vi "R-peak_detection_V2.vi"(9 "Cooldown in":i64, 10 "Threshold":dbl, 11 "ECG_vector":dbl[](array[numeric])) -> (1 "Cooldown out":i64, 3 "Rpeak_detected":bool)   [LabVIEW 2022 SP3]
uses:
  <vilib>/Analysis/NI_AALBase.lvlib
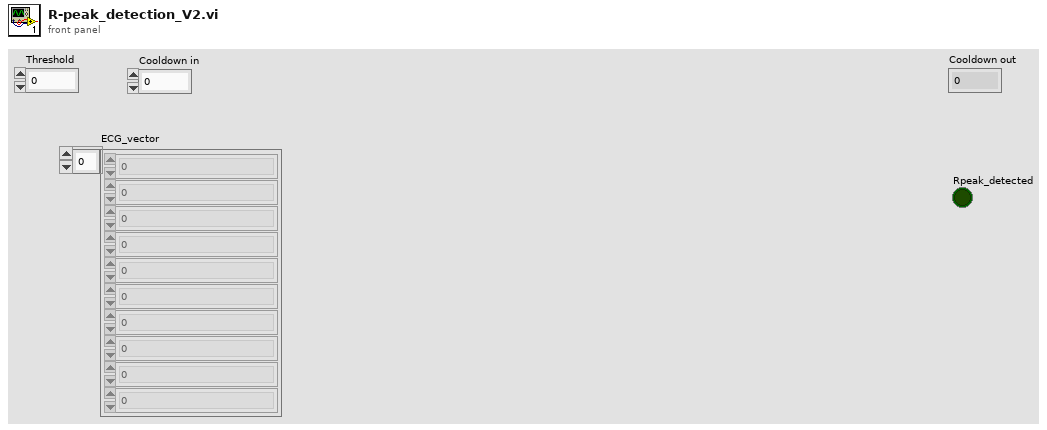
[diagram p1: front panel]
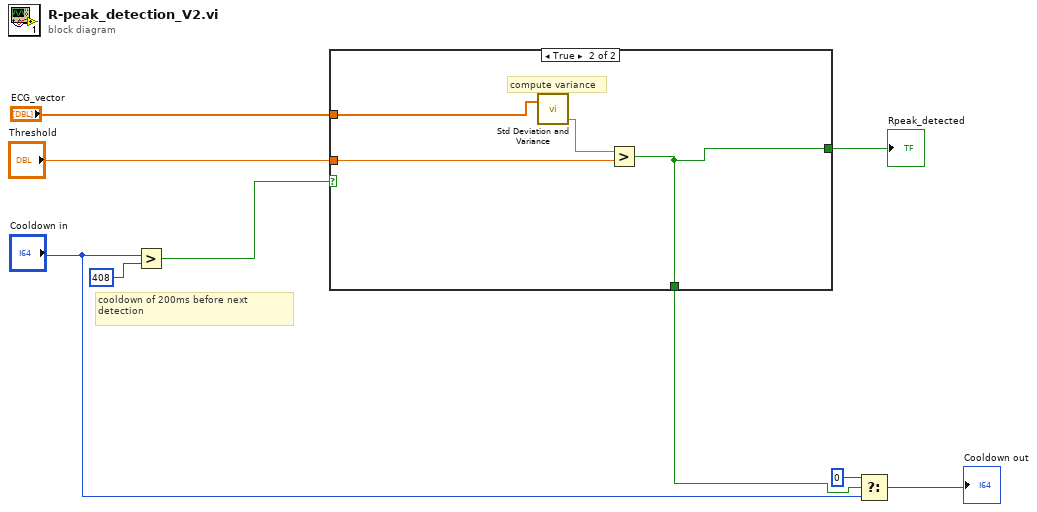
[diagram p0: block diagram]
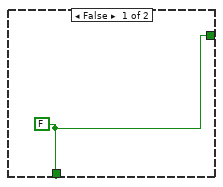
[diagram p2: hidden frame]
diagram:
  # "cooldown of 200ms before next detection"
  n1 = Greater?(x="Cooldown in", y=408) -> (0:w3:bool)
  n2 = case shown="True" w3 {
    tunnel: "ECG_vector" -> [_ w14]
    tunnel: "Threshold" -> [_ w12]
    tunnel: [w10 w11] -> w2
    tunnel: [w10 w11] -> w1
    frame False {
      w10 = FALSE
    }
    frame True {
      # "compute variance"
      n3 = call <vilib>:"Std Deviation and Variance.vi"("X"=w14) -> ("variance"=w13:dbl)  [unwired: 1 in, 2 out]
      n4 = Greater?(x=w13, y=w12) -> (0:w11:bool)
    }
  }
  "Rpeak_detected" <- w1
  n5 = Select(t=0, s=w2, f="Cooldown in") -> (s? t:f=→"Cooldown out":i64)
